vi "generate freq out sweep table.vi"(6 "Step Up and Down":bool, 9 "Step Size":dbl format="%.2f", 10 "Finish Frequency":dbl format="%.2f", 11 "Start Frequency":dbl format="%.2f") -> (2 "Clock, ClockDivisor, FreqDivisor, Frequency":dbl[][](array[numeric]) format="%.2f")   [LabVIEW 2021]
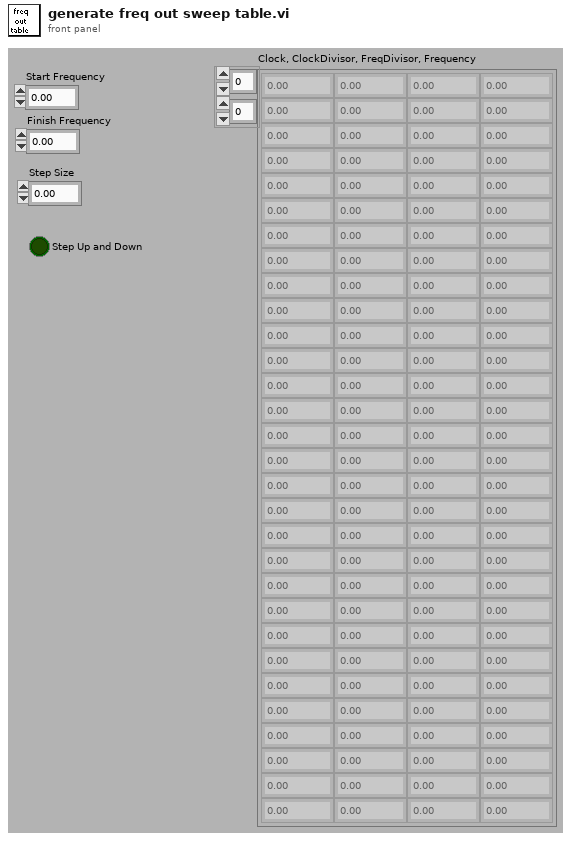
[diagram p1: front panel]
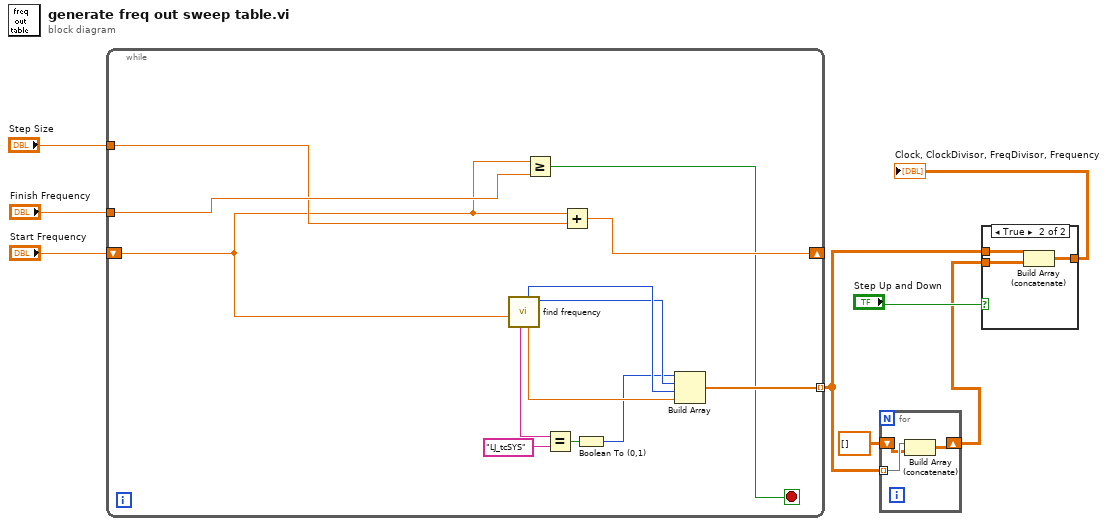
[diagram p0: block diagram]
diagram:
  n1 = while {
    tunnel: "Step Size" -> [w17]
    tunnel: "Finish Frequency" -> [w19]
    tunnel: [w21] -> w3 mode=indexing
    shift-left: "Start Frequency" -> [w13]
    shift-right: [w20] -> _
    stop <- w18 stop-if-true
    n2 = call "find frequency.vi"("target frequency"=w13) -> ("ClockDivisor"=w15:i32, "Frequency"=w14:dbl, "FreqDivisor"=w16:i32, "Clock Source"=w12:string)  [unwired: 5 in, 2 out]
    n3 = Greater Or Equal?(x=w13, y=w19) -> (x >= y?=w18:bool)
    n4 = Equal?(x=w12, y="LJ_tcSYS") -> (x = y?=w11:bool)
    n5 = Add(x=w13, y=w17) -> (x+y=w20:dbl)
    n6 = Boolean To (0,1)(Boolean=w11) -> (0, 1=w9:i16)
    n7 = Build Array(w9, w15, w16, w14) -> (w21:dbl[])
  }
  n8 = for {
    tunnel: w3 -> [w24] mode=indexing
    shift-right: [w22] -> w1
    shift-left: dbl[][] [] -> [w23]
    n9 = Build Array (concatenate)(w24, w23) -> (w22:dbl[][])
  }
  n10 = case shown="True" "Step Up and Down" {
    tunnel: w1 -> [_ w28]
    tunnel: w3 -> [w25 w27]
    tunnel: [w25 w26] -> w2
    frame False {
    }
    frame True {
      n11 = Build Array (concatenate)(w27, w28) -> (w26:dbl[][])
    }
  }
  "Clock, ClockDivisor, FreqDivisor, Frequency" <- w2
